vi "chmHelper.vi"(8 "error in (no error)":errorcluster, 9 "HTML File":string="MainPage_J1939.html", 10 "Main CHM File":string="J1939.chm", 11 "Automation Refnum in":refnum<k7>(container)) -> (0 "error out":errorcluster)   [LabVIEW 2020, in "Vires VTD System Explorer.lvlib"]
uses:
  Vires VTD System Explorer.lvlib
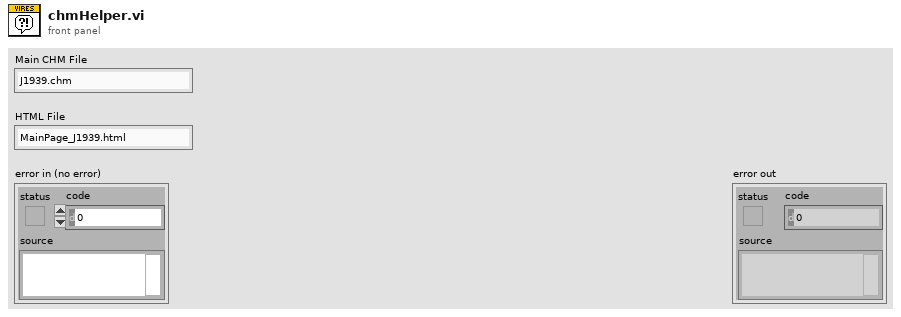
[diagram p1: front panel]
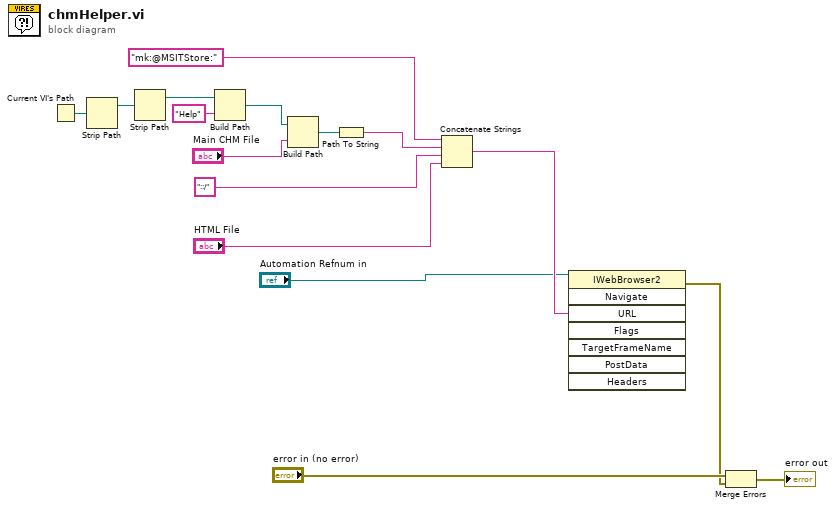
[diagram p0: block diagram]
diagram:
  n1 = Current VI's Path() -> (path=w10:path)
  n2 = Strip Path(path=w10) -> (stripped path=w11:path)  [unwired: 1 out]
  n3 = Strip Path(path=w11) -> (stripped path=w14:path)  [unwired: 1 out]
  n4 = Build Path(base path=w14, name or relative path="Help") -> (appended path=w3:path)
  n5 = Build Path(base path=w3, name or relative path="Main CHM File") -> (appended path=w1:path)
  n6 = Path To String(path=w1) -> (string=w13:string)
  n7 = Concatenate Strings("mk:@MSITStore:" ("string"), w13, "::/" ("name or relative path"), "HTML File") -> (w16:string)
  n8 = invoke class="IWebBrowser2" method="Navigate"(reference="Automation Refnum in", "URL"=w16) -> (error out=w6:errorcluster)  [unwired: 6 in, 7 out]
  n9 = Merge Errors("error in (no error)", w6) -> (→"error out":errorcluster)
